vi "Synthetic_Jet_LDA.vi"() -> (5 "Plug in titles":string[](array[string]), 7 "Plug in values":string[](array[string]))   [LabVIEW 2011]
uses:
  Controls/SJ_Data_Cluster.ctl
  Controls/SJ_Results_Cluster.ctl
  Controls/SJ_Channels.ctl
  Globals/Meas_global.vi
  <vilib>/Analysis/1siggen.llb/Ramp Pattern by Delta.vi
  <vilib>/Analysis/NI_AALBase.lvlib
  <vilib>/gmath/NI_Gmath.lvlib
  <vilib>/Analysis/NI_AALPro.lvlib
panel:
  out "Data Array":dbl[][](array[numeric])
  out "ALL filepath":path
  out "File Paths":path[][](array[path])
  out "Channel Varaibles":string[](array[string])
  out "Variable Names":string[](array[string])
  out "Target Frequency":dbl
  out "Results Folder Exists?":bool
  out "SJ Results Array":T1[](array[typedef])
  out "Dwell Time":u32=200
  out "No of Analogue Samples":i32=40000
  out "Analogue Aquisition Time":dbl=999.975
  out "Analogue Samples":i32=39999
  out "dt":dbl=inf
  out "No of bins":i32
  out "Analogue Fs":dbl=40000.0
  out "Next Frequency":dbl=1060.0
  out "Zero Values":dbl[](array[numeric])=[0.0030001498508715582, 0.0061511235517187676, 2.208881239967972, 0.0008108304920773175, 1.5203627177178738]
  out "SJ Data":T2={"Do"=0.005, "Dc"=0.038, "Ho"=0.01, "Hc"=0.008, "K"=1.14, "beta"=0.424, "Vc"=2.0, "Vo"=2.375}
  out "Current Frequency":dbl=1039.7638647645044 format="%0.4f"
  out "Frequency Array":dbl[](array[numeric])=[600.0, 620.0, 640.0, 660.0, 680.0, 700.0, 720.0, 740.0, 760.0, 780.0, 800.0, 820.0, 840.0, 860.0, 880.0, 900.0, 920.0, 940.0, 960.0, 980.0, 1000.0, 1020.0, 1040.0, 1060.0, 1080.0, 1100.0, 1120.0, 1140.0, 1160.0, 1180.0, 1200.0]
  # "You Must have selected the \"Save Data\" option on the \nMeasurement Program for this vi to work correctly"
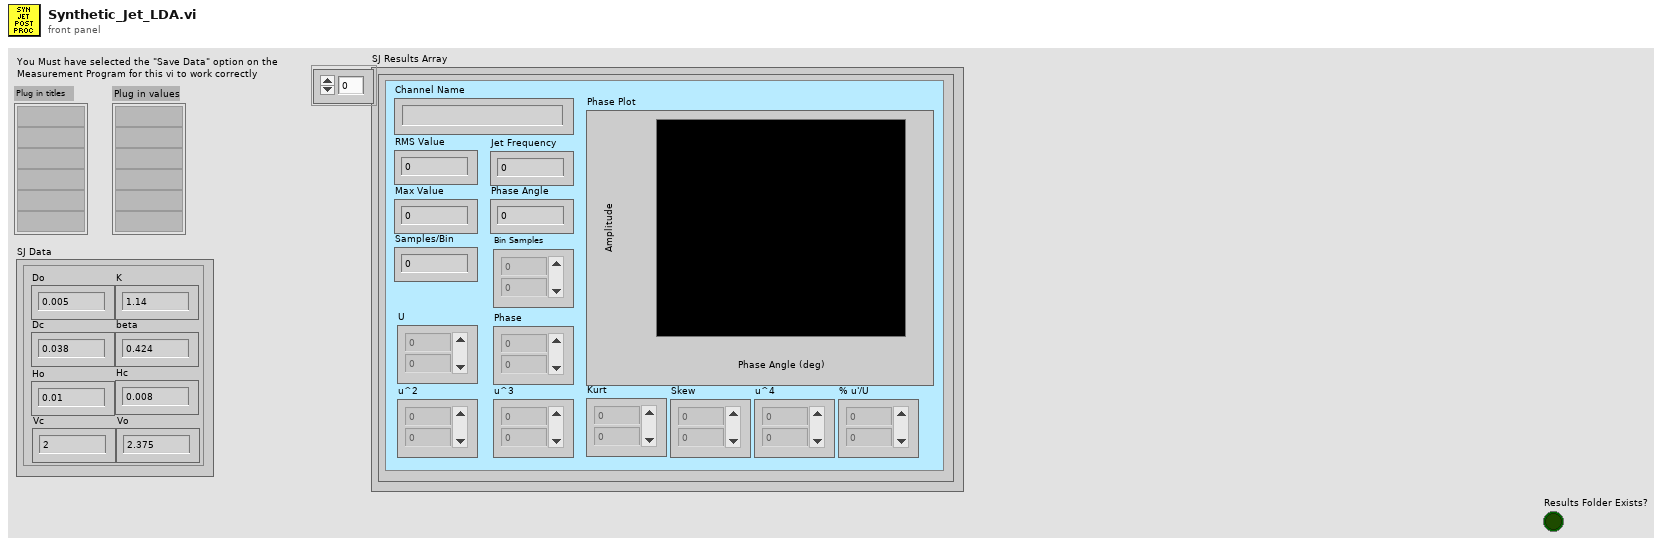
[diagram p1: front panel]
types:
  T1 = typedef "SJ_Results_Cluster.ctl" = cluster{"U":dbl[], "u^2":dbl[], "u^3":dbl[], "u^4":dbl[], "Skew":dbl[], "Kurt":dbl[], "% u'/U":dbl[], "Phase":dbl[], "Bin Samples":dbl[], "Phase Plot":cluster{"Phase Angle":dbl[], dbl[]}, "Channel Name":string, "Max Value":dbl, "RMS Value":dbl, "Phase Angle":dbl, "Jet Frequency":dbl, "Samples/Bin":i32}
  T2 = typedef "SJ_Data_Cluster.ctl" = cluster{"Do":dbl, "Dc":dbl, "Ho":dbl, "Hc":dbl, "K":dbl, "beta":dbl, "Vc":dbl, "Vo":dbl}
  T3 = typedef "SJ_Channels.ctl" = string[]
  T4 = typedef "Analysis_info_cluster.ctl" = cluster{"Colour":u32, "Inst type":T5, "Inst name":string, "Symbol":string, "Code name":string, "Extra Info":string, "Inst Array":T6, "Index":i32, "Voltage Index":i32, "Extra Titles":string[], "Extra Values":string[], "Eng Values":dbl[], "Time (ms)":dbl[], "TT / Voltage":dbl[], "U":dbl, "u^2":dbl, "u^3":dbl, "u^4":dbl, "Skew_u":dbl, "Kurt_u":dbl, "Mean % Err":dbl, "% u'/U":dbl}
  T5 = typedef "Inst_type.ctl" = enum16{"Propeller anemometer", "Raw voltage", "Pressure Transducer", "Pitot-static tube", "Preston tube", "Hot wire", "Cross wire 1", "Cross wire 2", "Generic Linear", "Generic Polynomial", "Generic BackPoly", "Fast FID", "Thermocouple", "Cold wire", "Pulsed Wire", "LDA Vel", "LDA Tran time", "LDA Arr time"}
  T6 = typedef "Instrument_Array.ctl" = enum16{"PWA", "LDA", "Analogue"}
  T7 = typedef "Post_Process.ctl" = enum16{"Take New Data", "Post Process Raw Data File"}
  T8 = cluster{"Name":string, "X":dbl, "Y":dbl, "Z":dbl}[]
  T9 = cluster{"Name":string, "X":dbl, "Y":dbl, "Z":dbl}
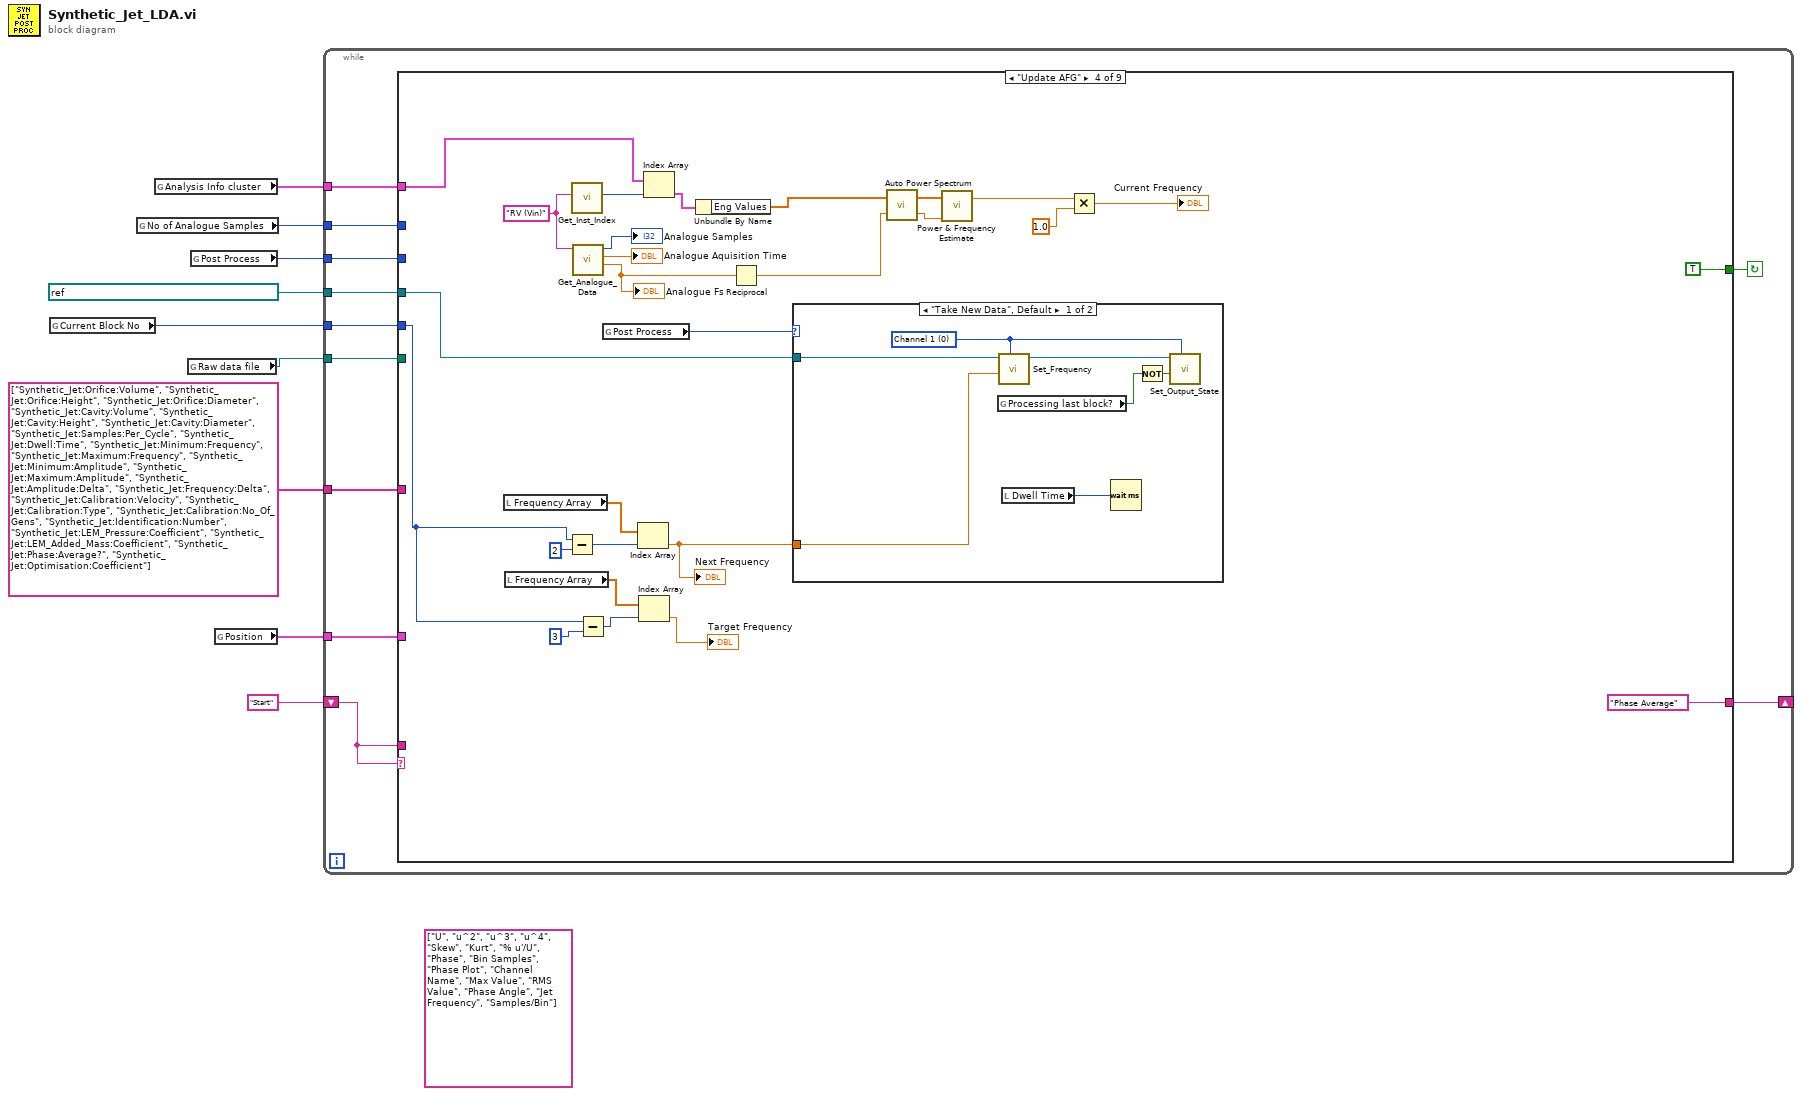
[diagram p0: block diagram]
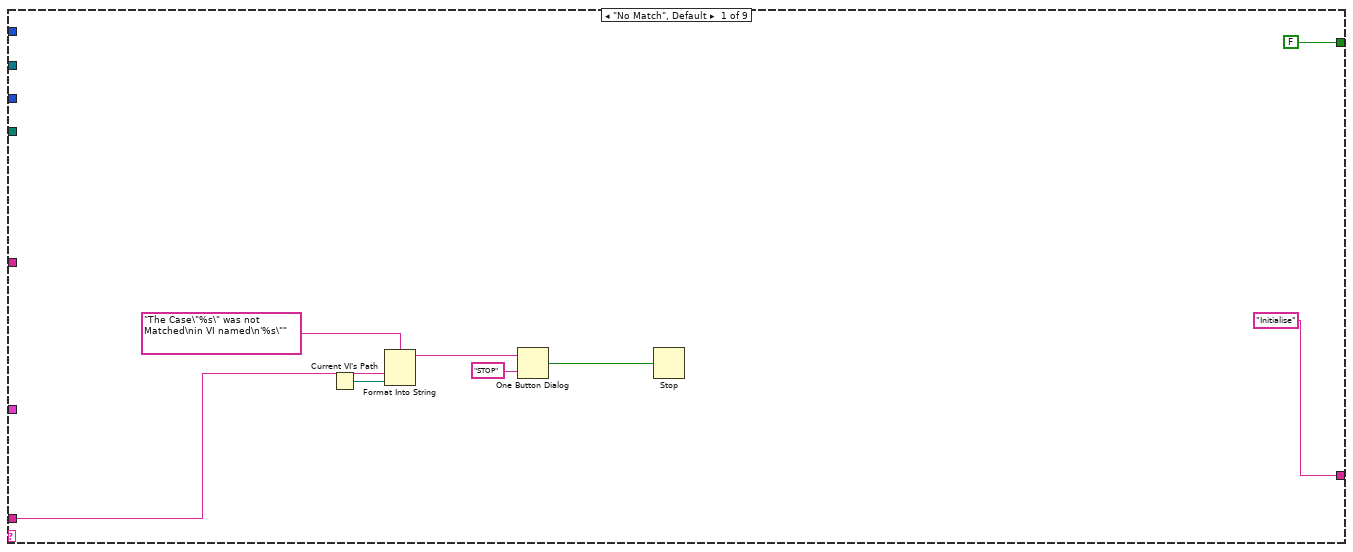
[diagram p2: hidden frame]
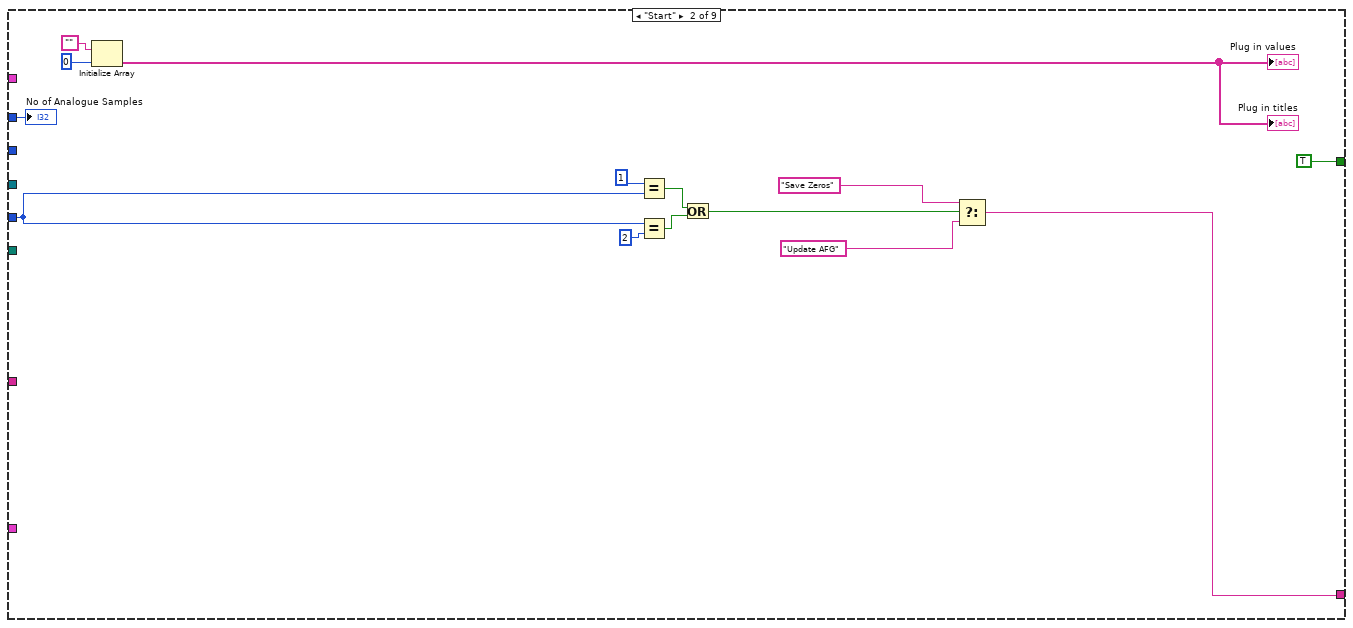
[diagram p3: hidden frame]
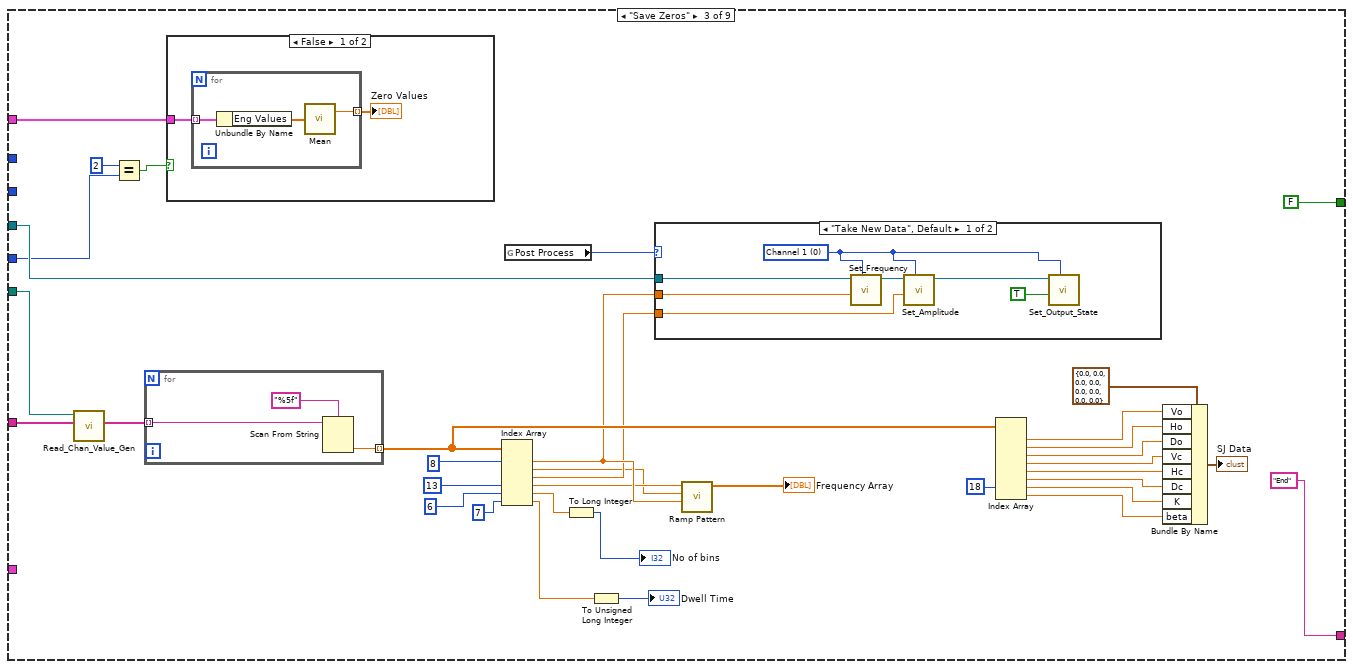
[diagram p4: hidden frame]
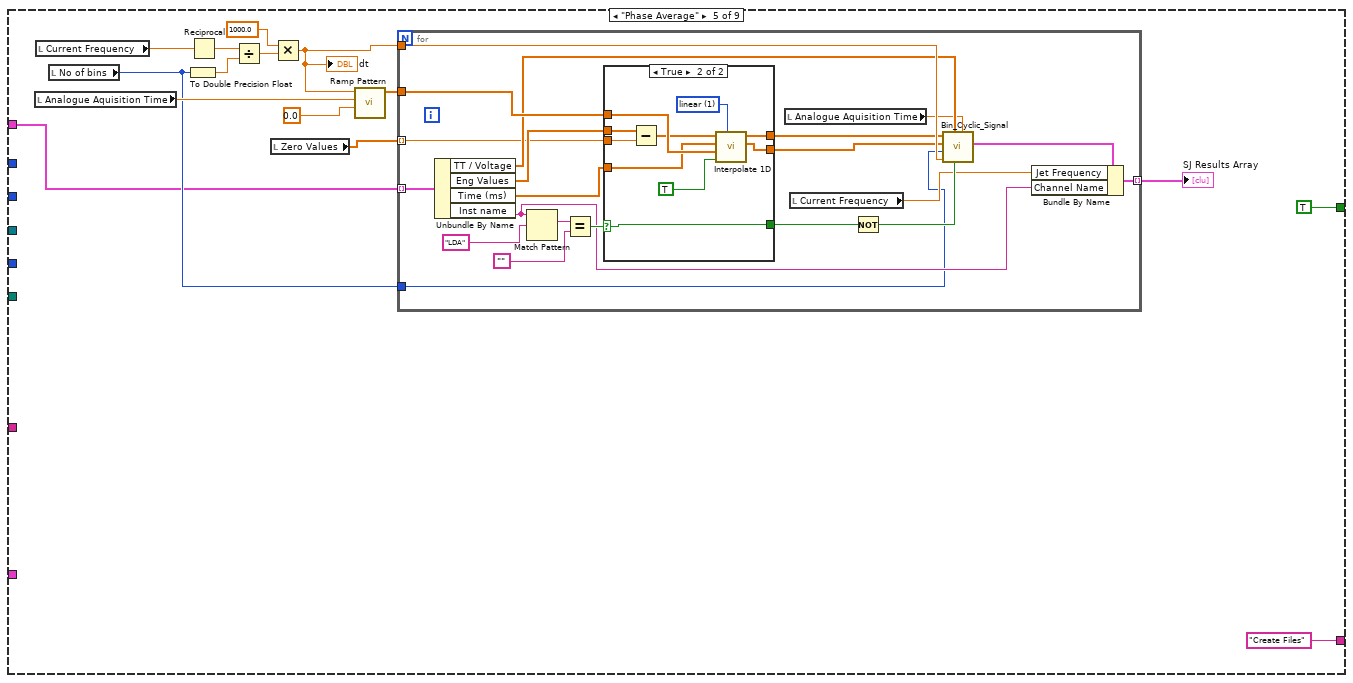
[diagram p8: hidden frame]
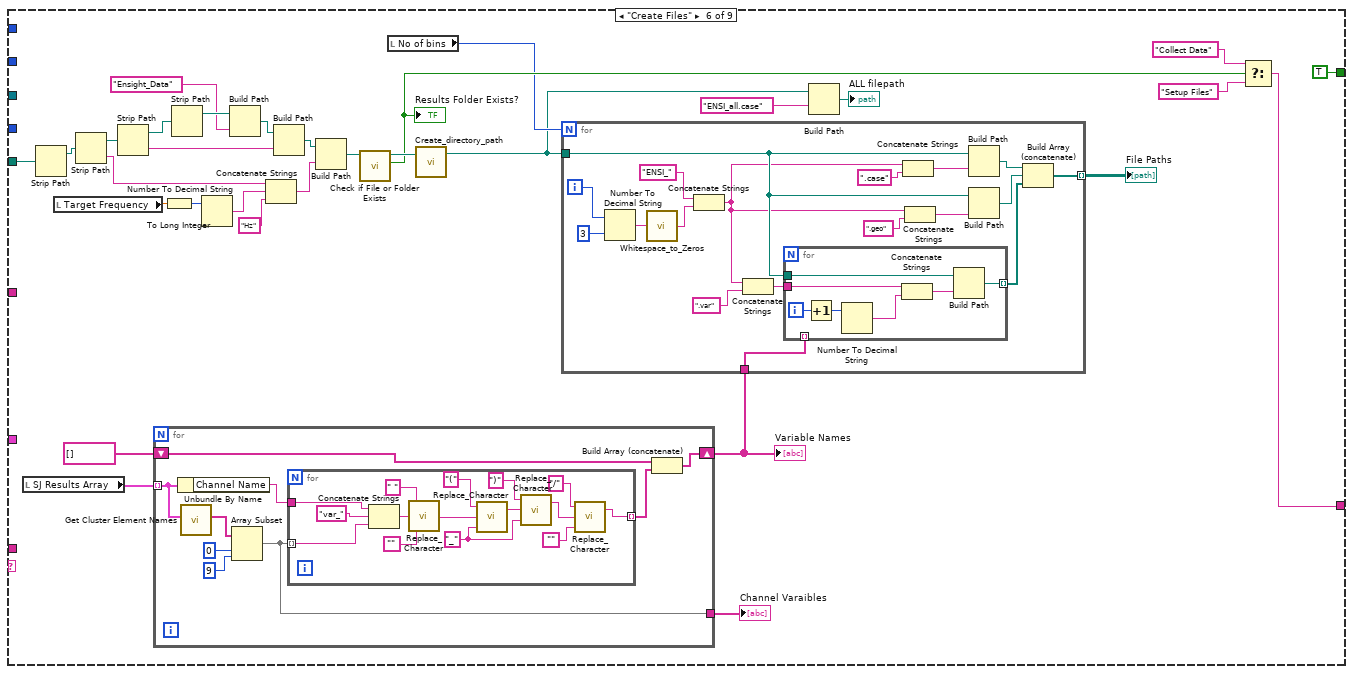
[diagram p10: hidden frame]
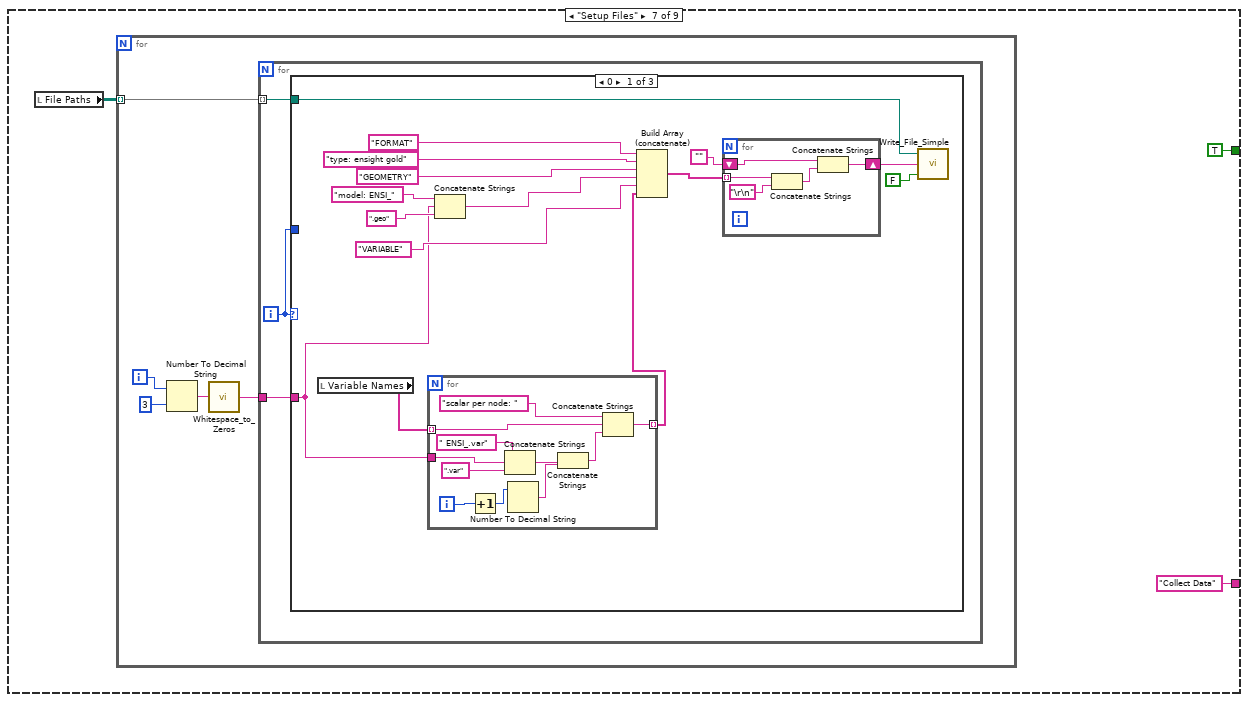
[diagram p11: hidden frame]
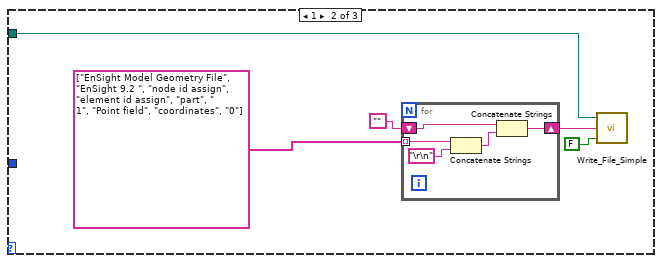
[diagram p12: hidden frame]
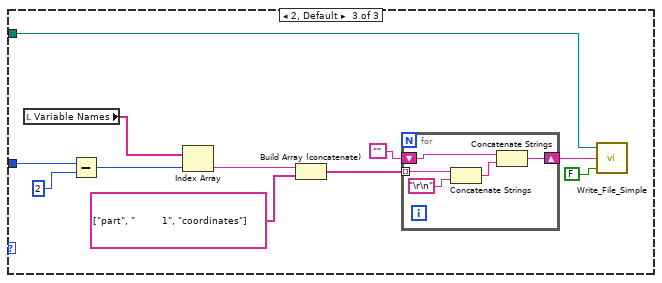
[diagram p13: hidden frame]
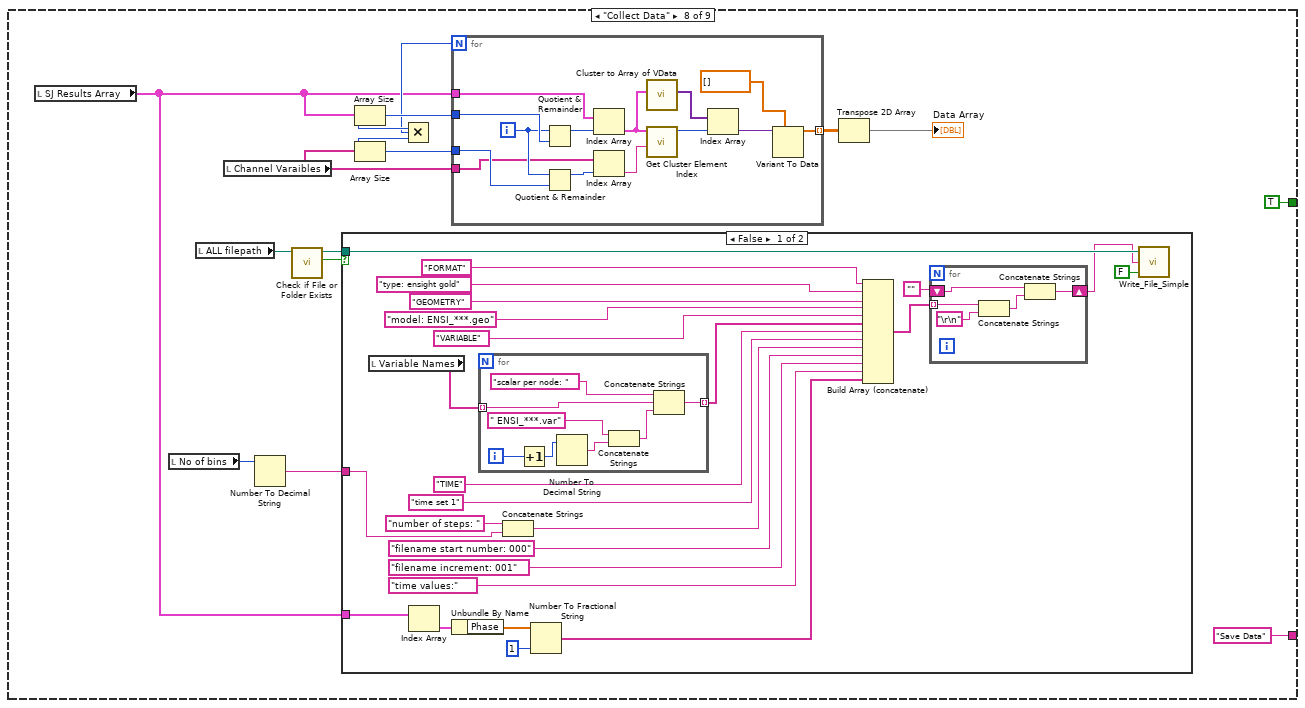
[diagram p14: hidden frame]
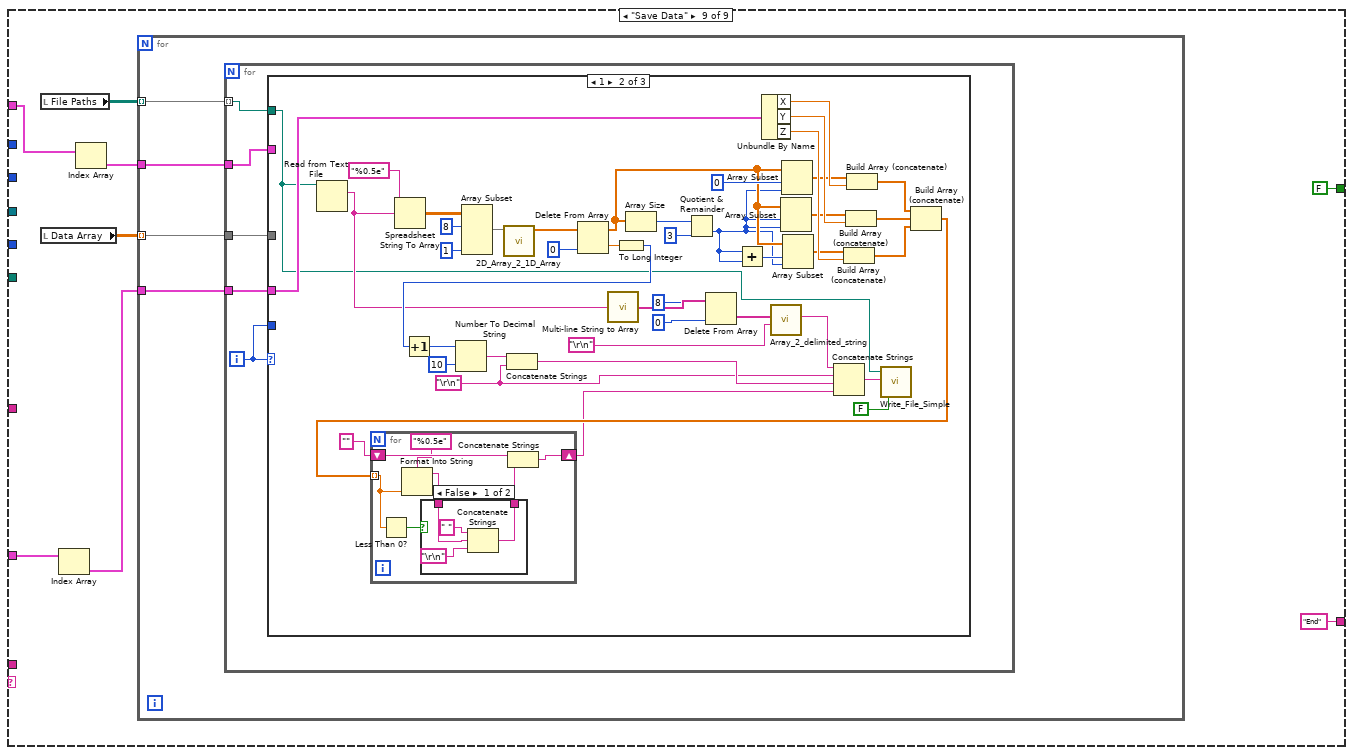
[diagram p16: hidden frame]
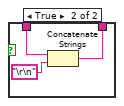
[diagram p18: hidden frame]
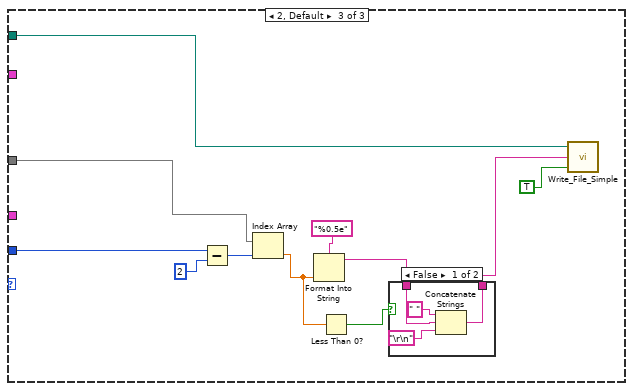
[diagram p19: hidden frame]
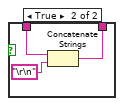
[diagram p20: hidden frame]
diagram:
  (unwired) string[] ["U", "u^2", "u^3", "u^4", "Skew", "Kurt", "% u'/U", "Phase", "Bin Samples", "Phase Plot", "Channel Name", "Max Value", "RMS Value", "Phase Angle", "Jet Frequency", "Samples/Bin"] ("Element Names")
  n1 = global read "Meas_global.vi" "Current Block No"() -> (w7:i32)
  n2 = global read "Meas_global.vi" "No of Analogue Samples"() -> (w5:i32)
  n3 = global read "Meas_global.vi" "Analysis Info cluster"() -> (w6:T4[])
  n4 = global read "Meas_global.vi" "Raw data file"() -> (w8:path)
  n5 = global read "Meas_global.vi" "Post Process"() -> (w3:T7)
  n6 = global read "Meas_global.vi" "Position"() -> (w4:T8)
  n7 = while {
    shift-left: "Start" -> [w20]
    shift-right: [w14] -> _
    tunnel: w8 -> [w19]
    tunnel: w7 -> [w15]
    tunnel: w6 -> [w18]
    tunnel: w5 -> [w17]
    tunnel: w4 -> [w16]
    tunnel: w3 -> [w12]
    tunnel: T3 ["Synthetic_Jet:Orifice:Volume", "Synthetic_Jet:Orifice:Height", "Synthetic_Jet:Orifice:Diameter", "Synthetic_Jet:Cavity:Volume", "Synthetic_Jet:Cavity:Height", "Synthetic_Jet:Cavity:Diameter", "Synthetic_Jet:Samples:Per_Cycle", "Synthetic_Jet:Dwell:Time", "Synthetic_Jet:Minimum:Frequency", "Synthetic_Jet:Maximum:Frequency", "Synthetic_Jet:Minimum:Amplitude", "Synthetic_Jet:Maximum:Amplitude", "Synthetic_Jet:Amplitude:Delta", "Synthetic_Jet:Frequency:Delta", "Synthetic_Jet:Calibration:Velocity", "Synthetic_Jet:Calibration:Type", "Synthetic_Jet:Calibration:No_Of_Gens", "Synthetic_Jet:Identification:Number", "Synthetic_Jet:LEM_Pressure:Coefficient", "Synthetic_Jet:LEM_Added_Mass:Coefficient", "Synthetic_Jet:Phase:Average?", "Synthetic_Jet:Optimisation:Coefficient"] ("Synthetic Jet Specific Channels") -> [w11]
    tunnel: refnum<visa-resource-name> "USB0::0x0699::0x0347::C036837::INSTR" ("VISA resource name") -> [w10]
    stop <- w13 continue-if-true
    n8 = case shown="\"Update AFG\"" w20 {
      tunnel: w20 -> [w24 _ _ _ _ _ _ _ _]
      tunnel: w19 -> [_ _ w75 _ _ w196 _ _ _]
      tunnel: w15 -> [_ w34 w52 w103 _ _ _ _ _]
      tunnel: w18 -> [_ _ w54 w111 w130 _ _ _ w392]
      tunnel: w17 -> [_ w29 _ _ _ _ _ _ _]
      tunnel: w16 -> [_ _ _ _ _ _ _ _ w395]
      tunnel: ["Initialise" w39 "End" ("t") "Phase Average" ("t") "Create Files" ("t") w183 "Collect Data" ("t") "Save Data" ("t") "End" ("t")] -> w14
      tunnel: [FALSE TRUE FALSE TRUE TRUE TRUE TRUE TRUE FALSE] -> w13
      tunnel: w12 -> [_ _ _ _ _ _ _ _ _]
      tunnel: w11 -> [_ _ w74 _ _ _ _ _ _]
      tunnel: w10 -> [_ _ w60 w114 _ _ _ _ _]
      frame "No Match", Default {
        n9 = Current VI's Path() -> (path=w23:path)
        n10 = Format Into String(format string="The Case\"%s\" was not Matched\nin VI named\n'%s\"" ("Format String"), w24, w23) -> (resulting string=w27:string)  [unwired: 2 in, 1 out]
        n11 = One Button Dialog(message=w27, button name ("OK")="STOP") -> (true=w25:bool)
        n12 = Stop(stop? (T)=w25) -> ()
      }
      frame "Start" {
        n13 = Initialize Array("", 0) -> (→"Plug in values" →"Plug in titles":string[])
        n14 = Equal?(x=1, y=w34) -> (x = y?=w32:bool)
        n15 = Equal?(x=w34, y=2 ("x")) -> (x = y?=w33:bool)
        n16 = Or(x=w32, y=w33) -> (x .or. y?=w31:bool)
        n17 = Select(t="Save Zeros", s=w31, f="Update AFG") -> (s? t:f=w39:string)
        "No of Analogue Samples" <- w29
      }
      frame "Save Zeros" {
        n18 = call "Read_Chan_Value_Gen.vi"("Desired Ch Names"=w74, "Raw data file"=w75) -> ("Values"=w64:string[])  [unwired: 9 in]
        n19 = Equal?(x=2, y=w52) -> (x = y?=w50:bool)
        n20 = for {
          tunnel: w64 -> [w93] mode=indexing
          tunnel: [w91] -> w59 mode=indexing
          n21 = Scan From String(format string="%5f", input string=w93) -> (output 1=w91:dbl)  [unwired: 3 in, 3 out]
        }
        n22 = case shown="False" w50 {
          tunnel: w54 -> [w80 _]
          frame False {
            n23 = for {
              tunnel: w80 -> [w83] mode=indexing
              tunnel: [w81] -> w79 mode=indexing
              n24 = Unbundle By Name(w83) -> ("Eng Values"=w82:dbl[])
              n25 = call <vilib>:"Mean.vi"("X"=w82) -> ("mean"=w81:dbl)  [unwired: 1 out]
            }
            "Zero Values" <- w79
          }
          frame True {
          }
        }
        n26 = Index Array(array=w59, index #1=8 ("index"), index #4=13 ("index"), index #5=6 ("index"), index #6=7 ("index")) -> (element #1=w58:dbl, element #2=w49:dbl, element #3=w57:dbl, element #4=w56:dbl, element #5=w47:dbl, element #6=w45:dbl)  [unwired: 2 in]
        n27 = global read "Meas_global.vi" "Post Process"() -> (w61:T7)
        n28 = To Long Integer(number=w47) -> (32bit integer=→"No of bins":i32)
        n29 = To Unsigned Long Integer(number=w45) -> (unsigned 32bit integer=→"Dwell Time":u32)
        n30 = case shown="\"Take New Data\", Default" w61 {
          tunnel: w57 -> [w90 _]
          tunnel: w58 -> [w85 _]
          tunnel: w60 -> [w84 _]
          frame "Take New Data", Default {
            w87 = u16 0 items=["Channel 1", "Channel 2"] ("Menu Ring")
            n31 = call "Set_Frequency.vi"("Menu Ring"=w87, "Frequency"=w85, "VISA resource name"=w84) -> ("VISA resource name out"=w88:refnum<visa-resource-name>)  [unwired: 8 in]
            n32 = call "Set_Amplitude.vi"("Menu Ring 2"=w87, "Amplitude"=w90, "VISA resource name"=w88) -> ("VISA resource name out"=w89:refnum<visa-resource-name>)  [unwired: 8 in]
            n33 = call "Set_Output_State.vi"("Menu Ring"=w87, "Output State"=TRUE, "VISA resource name"=w89) -> ()  [unwired: 9 in]
          }
          frame "Post Process Raw Data File" {
          }
        }
        n34 = call-poly <vilib>:"Ramp Pattern.vi"("start"=w58, "end"=w49, "delta"=w56) -> ("Ramp Pattern"=→"Frequency Array":dbl[])  [unwired: 6 in, 2 out]
        n35 = Index Array(array=w59, index #7=18 ("index")) -> (element #1=w73:dbl, element #2=w72:dbl, element #3=w71:dbl, element #4=w70:dbl, element #5=w69:dbl, element #6=w68:dbl, element #7=w66:dbl, element #8=w65:dbl)  [unwired: 7 in]
        n36 = Bundle By Name(cluster=T2 {"Do"=0.0, "Dc"=0.0, "Ho"=0.0, "Hc"=0.0, "K"=0.0, "beta"=0.0, "Vc"=0.0, "Vo"=0.0} ("SJ_Data_Cluster"), "Vo"=w73, "Ho"=w72, "Do"=w71, "Vc"=w70, "Hc"=w69, "Dc"=w68, "K"=w66, "beta"=w65) -> (→"SJ Data":T2)
      }
      frame "Update AFG" {
        w112 = "RV (Vin)" ("Inst name search")
        n37 = local read "Frequency Array"() -> (w119:dbl[])
        n38 = local read "Frequency Array"() -> (w104:dbl[])
        n39 = Subtract(x=w103, y=2) -> (x-y=w118:i32)
        n40 = call "Get_Inst_Index.vi"("Inst name search"=w112) -> ("Index of Instance"=w110:i32)  [unwired: 8 in, 2 out]
        n41 = call "Get_Analogue_Data.vi"("Inst (Inst 2 if blank)"=w112) -> ("Analogue Fs"=w96:dbl, "Analogue Aquasition Time"=→"Analogue Aquisition Time":dbl, "Analogue Samples"=→"Analogue Samples":i32)  [unwired: 8 in]
        "Analogue Fs" <- w96
        n42 = Subtract(x=w103, y=3) -> (x-y=w101:i32)
        n43 = global read "Meas_global.vi" "Post Process"() -> (w115:T7)
        n44 = Index Array(array=w119, index=w118) -> (element=w116:dbl)
        "Next Frequency" <- w116
        n45 = Index Array(array=w104, index=w101) -> (element=→"Target Frequency":dbl)
        n46 = Index Array(array=w111, index=w110) -> (element=w109:T4)
        n47 = Unbundle By Name(w109) -> ("Eng Values"=w94:dbl[])
        n48 = Reciprocal(x=w96) -> (1/x=w95:dbl)
        n49 = case shown="\"Take New Data\", Default" w115 {
          tunnel: w116 -> [w126 _]
          tunnel: w114 -> [w124 _]
          frame "Take New Data", Default {
            w127 = u16 0 items=["Channel 1", "Channel 2"] ("Menu Ring")
            n50 = global read "Meas_global.vi" "Processing last block?"() -> (w122:bool)
            n51 = call "Set_Frequency.vi"("Menu Ring"=w127, "Frequency"=w126, "VISA resource name"=w124) -> ("VISA resource name out"=w125:refnum<visa-resource-name>)  [unwired: 8 in]
            n52 = local read "Dwell Time"() -> (w121:u32)
            n53 = Wait (ms)(milliseconds to wait=w121) -> ()  [unwired: 1 out]
            n54 = Not(x=w122) -> (.not. x?=w123:bool)
            n55 = call "Set_Output_State.vi"("Menu Ring"=w127, "Output State"=w123, "VISA resource name"=w125) -> ()  [unwired: 9 in]
          }
          frame "Post Process Raw Data File" {
          }
        }
        n56 = call <vilib>:"Auto Power Spectrum.vi"("dt"=w95, "Signal (V)"=w94) -> ("df"=w98:dbl, "Power Spectrum (V^2 rms)"=w97:dbl[])
        n57 = call <vilib>:"Power & Frequency Estimate.vi"("df"=w98, "Power Spectrum (V^2 rms)"=w97) -> ("est frequency peak"=w99:dbl)  [unwired: 4 in, 1 out]
        n58 = Multiply(x=w99, y=1.0) -> (x*y=→"Current Frequency":dbl)
      }
      frame "Phase Average" {
        n59 = local read "Analogue Aquisition Time"() -> (w137:dbl)
        n60 = local read "Current Frequency"() -> (w134:dbl)
        n61 = local read "No of bins"() -> (w131:i32)
        n62 = To Double Precision Float(number=w131) -> (double precision float=w140:dbl)
        n63 = Reciprocal(x=w134) -> (1/x=w139:dbl)
        n64 = Divide(x=w139, y=w140) -> (x/y=w136:dbl)
        n65 = local read "Zero Values"() -> (w129:dbl[])
        n66 = Multiply(x=1000.0, y=w136) -> (x*y=w132:dbl)
        "dt" <- w132
        n67 = call-poly <vilib>:"Ramp Pattern.vi"("start"=0.0, "end"=w137, "delta"=w132) -> ("Ramp Pattern"=w133:dbl[])  [unwired: 6 in, 2 out]
        n68 = for {
          tunnel: w133 -> [w163]
          tunnel: w132 -> [w162]
          tunnel: w131 -> [w147]
          tunnel: w130 -> [w145] mode=indexing
          tunnel: w129 -> [w144] mode=indexing
          tunnel: [w143] -> w128 mode=indexing
          n69 = Unbundle By Name(w145) -> ("TT / Voltage"=w152:dbl[], "Eng Values"=w156:dbl[], "Time (ms)"=w157:dbl[], "Inst name"=w149:string)
          n70 = Match Pattern(string=w149, regular expression="LDA") -> (match substring=w160:string)  [unwired: 1 in, 3 out]
          n71 = Equal?(x=w160, y="") -> (x = y?=w158:bool)
          n72 = case shown="True" w158 {
            selector: w158 -> [w164 w170]
            tunnel: w163 -> [_ w175]
            tunnel: w157 -> [w165 w174]
            tunnel: w156 -> [w166 w169]
            tunnel: [w166 w172] -> w146
            tunnel: [w165 w171] -> w155
            tunnel: [w164 w170] -> w154
            tunnel: w144 -> [_ w167]
            frame False {
            }
            frame True {
              w176 = 1 items=["nearest", "linear", "spline", "cubic Hermite", "Lagrange"] ("method")
              n73 = Subtract(x=w169, y=w167) -> (x-y=w168:dbl[])
              n74 = call <vilib>:"Interpolate 1D.vi"("method"=w176, "X is monotonic"=TRUE, "xi"=w175, "X"=w174, "Y"=w168) -> ("xi used"=w171:dbl[], "yi"=w172:dbl[])  [unwired: 4 in, 1 out]
            }
          }
          n75 = local read "Analogue Aquisition Time"() -> (w151:dbl)
          n76 = local read "Current Frequency"() -> (w148:dbl)
          n77 = Not(x=w154) -> (.not. x?=w153:bool)
          n78 = call "Bin_Cyclic_Signal.vi"("Max Time"=w151, "LDA Data? (False)"=w153, "Transit Time"=w152, "dt"=w162, "No of bins"=w147, "Time"=w155, "Eng Values"=w146) -> ("SJ Results"=w150:T1)  [unwired: 4 in]
          n79 = Bundle By Name(cluster=w150, "Jet Frequency"=w148, "Channel Name"=w149) -> (w143:T1)
        }
        "SJ Results Array" <- w128
      }
      frame "Create Files" {
        n80 = local read "SJ Results Array"() -> (w179:T1[])
        n81 = Strip Path(path=w196) -> (stripped path=w206:path)  [unwired: 1 out]
        n82 = local read "Target Frequency"() -> (w195:dbl)
        n83 = Strip Path(path=w206) -> (stripped path=w205:path, name=w193:string)
        n84 = Strip Path(path=w205) -> (stripped path=w204:path, name=w200:string)
        n85 = for {
          tunnel: w179 -> [w233] mode=indexing
          shift-right: [w237] -> w188
          shift-left: string[] [] -> [w235]
          tunnel: [w234] -> w187
          n86 = Unbundle By Name(w233) -> ("Channel Name"=w238:string)
          n87 = call "Get Cluster Element Names.vi"("Cluster"=w233) -> ("Element Names"=w241:string[])  [unwired: 9 in, 1 out]
          n88 = Array Subset(array=w241, index=0, length=9) -> (w234:string[])
          n89 = for {
            tunnel: w234 -> [w256] mode=indexing
            tunnel: w238 -> [w255]
            tunnel: [w243] -> w236 mode=indexing
            w247 = "_" ("Replace with")
            n90 = Concatenate Strings(w255, "var_" ("string"), w256) -> (w253:string)
            n91 = call "Replace_Character.vi"("Replace with"="", "Input String"=w253, "Search For"=" ") -> ("Output string"=w242:string)  [unwired: 1 out]
            n92 = call "Replace_Character.vi"("Replace with"=w247, "Input String"=w242, "Search For"="(") -> ("Output string"=w249:string)  [unwired: 1 out]
            n93 = call "Replace_Character.vi"("Replace with"=w247, "Input String"=w249, "Search For"=")") -> ("Output string"=w246:string)  [unwired: 1 out]
            n94 = call "Replace_Character.vi"("Replace with"="", "Input String"=w246, "Search For"="/") -> ("Output string"=w243:string)  [unwired: 1 out]
          }
          n95 = Build Array (concatenate)(w235, w236) -> (w237:string[])
        }
        "Variable Names" <- w188
        "Channel Varaibles" <- w187
        n96 = To Long Integer(number=w195) -> (32bit integer=w194:i32)
        n97 = Strip Path(path=w204) -> (stripped path=w203:path)  [unwired: 1 out]
        n98 = Number To Decimal String(number=w194) -> (decimal integer string=w192:string)  [unwired: 1 in]
        n99 = Build Path(base path=w203, name or relative path="Ensight_Data") -> (appended path=w201:path)
        n100 = Concatenate Strings(w193, w192, "Hz" ("string")) -> (w190:string)
        n101 = Build Path(base path=w201, name or relative path=w200) -> (appended path=w197:path)
        n102 = Build Path(base path=w197, name or relative path=w190) -> (appended path=w198:path)
        n103 = call <vilib>:"Check if File or Folder Exists.vi"("path"=w198) -> ("file or folder exists?"=w184:bool, "dup path"=w199:path)  [unwired: 8 in, 1 out]
        "Results Folder Exists?" <- w184
        n104 = local read "No of bins"() -> (w182:i32)
        n105 = call "Create_directory_path.vi"("Path name"=w199) -> ("Path name Out"=w177:path)  [unwired: 1 in, 1 out]
        n106 = for {
          N: w182 -> [_]
          tunnel: w177 -> [w225]
          tunnel: w188 -> [w224]
          tunnel: [w223] -> w178 mode=indexing
          i -> [w219]
          n107 = Number To Decimal String(number=w219, width (-)=i16 3) -> (decimal integer string=w217:string)
          n108 = call "Whitespace_to_Zeros.vi"("Input String"=w217) -> ("Output String"=w213:string)  [unwired: 6 in]
          n109 = Concatenate Strings("ENSI_" ("name or relative path"), w213) -> (w209:string)
          n110 = Concatenate Strings(w209, ".var" ("name or relative path")) -> (w208:string)
          n111 = for {
            tunnel: w225 -> [w232]
            tunnel: [w227] -> w220 mode=indexing
            tunnel: w224 -> [_] mode=indexing
            tunnel: w208 -> [w226]
            i -> [w231]
            n112 = Increment(x=w231) -> (x+1=w230:i32)
            n113 = Number To Decimal String(number=w230) -> (decimal integer string=w229:string)  [unwired: 1 in]
            n114 = Concatenate Strings(w226, w229) -> (w228:string)
            n115 = Build Path(base path=w232, name or relative path=w228) -> (appended path=w227:path)
          }
          n116 = Concatenate Strings(w209, ".case" ("name or relative path")) -> (w216:string)
          n117 = Concatenate Strings(w209, ".geo" ("name or relative path")) -> (w212:string)
          n118 = Build Path(base path=w225, name or relative path=w216) -> (appended path=w221:path)
          n119 = Build Path(base path=w225, name or relative path=w212) -> (appended path=w222:path)
          n120 = Build Array (concatenate)(w221, w222, w220) -> (w223:path[])
        }
        "File Paths" <- w178
        n121 = Build Path(base path=w177, name or relative path="ENSI_all.case") -> (appended path=→"ALL filepath":path)
        n122 = Select(t="Collect Data", s=w184, f="Setup Files" ("t")) -> (s? t:f=w183:string)
      }
      frame "Setup Files" {
        n123 = local read "File Paths"() -> (w258:path[][])
        n124 = for {
          tunnel: w258 -> [w264] mode=indexing
          i -> [w261]
          n125 = Number To Decimal String(number=w261, width (-)=i16 3) -> (decimal integer string=w262:string)
          n126 = call "Whitespace_to_Zeros.vi"("Input String"=w262) -> ("Output String"=w260:string)  [unwired: 6 in]
          n127 = for {
            tunnel: w264 -> [w267] mode=indexing
            tunnel: w260 -> [w265]
            i -> [w266]
            n128 = case shown="0" w266 {
              tunnel: w267 -> [w278 w300 w319]
              tunnel: w266 -> [_ _ w314]
              tunnel: w265 -> [w268 _ _]
              frame 0 {
                n129 = local read "Variable Names"() -> (w282:string[])
                n130 = for {
                  tunnel: w282 -> [w294] mode=indexing
                  tunnel: [w292] -> w277 mode=indexing
                  tunnel: w268 -> [w289]
                  i -> [w296]
                  n131 = Increment(x=w296) -> (x+1=w297:i32)
                  n132 = Concatenate Strings(" ENSI_.var", w289, ".var") -> (w291:string)
                  n133 = Number To Decimal String(number=w297) -> (decimal integer string=w295:string)  [unwired: 1 in]
                  n134 = Concatenate Strings(w291, w295) -> (w293:string)
                  n135 = Concatenate Strings("scalar per node: ", w294, w293) -> (w292:string)
                }
                n136 = Concatenate Strings("model: ENSI_", w268, ".geo") -> (w270:string)
                n137 = Build Array (concatenate)("FORMAT", "type: ensight gold", "GEOMETRY", w270, "VARIABLE", w277) -> (w276:string[])
                n138 = for {
                  tunnel: w276 -> [w287] mode=indexing
                  shift-right: [w285] -> w280
                  shift-left: "" -> [w283]
                  n139 = Concatenate Strings(w287, "\r\n") -> (w284:string)
                  n140 = Concatenate Strings(w283, w284) -> (w285:string)
                }
                n141 = call "Write_File_Simple.vi"("append to file? (new file:F)"=FALSE, "character string"=w280, "file path"=w278) -> ()  [unwired: 2 out]
              }
              frame 1 {
                n142 = for {
                  tunnel: string[] ["EnSight Model Geometry File", "EnSight 9.2 ", "node id assign", "element id assign", "part", "         1", "Point field", "coordinates", "0"] -> [w308] mode=indexing
                  shift-right: [w306] -> w302
                  shift-left: "" -> [w304]
                  n143 = Concatenate Strings(w308, "\r\n") -> (w305:string)
                  n144 = Concatenate Strings(w304, w305) -> (w306:string)
                }
                n145 = call "Write_File_Simple.vi"("append to file? (new file:F)"=FALSE, "character string"=w302, "file path"=w300) -> ()  [unwired: 2 out]
              }
              frame 2, Default {
                n146 = local read "Variable Names"() -> (w315:string[])
                n147 = Subtract(x=w314, y=2) -> (x-y=w312:i32)
                n148 = Index Array(array=w315, index=w312) -> (element=w311:string)
                n149 = Build Array (concatenate)(w311, string[] ["part", "         1", "coordinates"]) -> (w309:string[])
                n150 = for {
                  tunnel: w309 -> [w324] mode=indexing
                  shift-right: [w322] -> w317
                  shift-left: "" -> [w320]
                  n151 = Concatenate Strings(w324, "\r\n") -> (w321:string)
                  n152 = Concatenate Strings(w320, w321) -> (w322:string)
                }
                n153 = call "Write_File_Simple.vi"("append to file? (new file:F)"=FALSE, "character string"=w317, "file path"=w319) -> ()  [unwired: 2 out]
              }
            }
          }
        }
      }
      frame "Collect Data" {
        n154 = local read "SJ Results Array"() -> (w327:T1[])
        n155 = local read "No of bins"() -> (w326:i32)
        n156 = local read "ALL filepath"() -> (w330:path)
        n157 = local read "Channel Varaibles"() -> (w335:string[])
        n158 = Number To Decimal String(number=w326) -> (decimal integer string=w325:string)  [unwired: 1 in]
        n159 = call <vilib>:"Check if File or Folder Exists.vi"("path"=w330) -> ("file or folder exists?"=w329:bool, "dup path"=w328:path)  [unwired: 8 in, 1 out]
        n160 = case shown="False" w329 {
          tunnel: w328 -> [w363 _]
          tunnel: w327 -> [w361 _]
          tunnel: w325 -> [w345 _]
          frame False {
            n161 = local read "Variable Names"() -> (w352:string[])
            n162 = Index Array(array=w361) -> (element=w360:T1)  [unwired: 1 in]
            n163 = Unbundle By Name(w360) -> ("Phase"=w359:dbl[])
            n164 = for {
              tunnel: w352 -> [w372] mode=indexing
              tunnel: [w370] -> w351 mode=indexing
              i -> [w374]
              n165 = Increment(x=w374) -> (x+1=w375:i32)
              n166 = Number To Decimal String(number=w375) -> (decimal integer string=w373:string)  [unwired: 1 in]
              n167 = Concatenate Strings(" ENSI_***.var", w373) -> (w371:string)
              n168 = Concatenate Strings("scalar per node: ", w372, w371) -> (w370:string)
            }
            n169 = Concatenate Strings("number of steps: ", w345) -> (w343:string)
            n170 = Number To Fractional String(number=w359, precision (6)=i16 1) -> (F-format string=w339:string[])  [unwired: 2 in]
            n171 = Build Array (concatenate)("FORMAT", "type: ensight gold", "GEOMETRY", "model: ENSI_***.geo", "VARIABLE", w351, "TIME", "time set 1", w343, "filename start number: 000", "filename increment: 001", "time values:", w339) -> (w348:string[])
            n172 = for {
              tunnel: w348 -> [w368] mode=indexing
              shift-right: [w366] -> w349
              shift-left: "" -> [w364]
              n173 = Concatenate Strings(w368, "\r\n") -> (w365:string)
              n174 = Concatenate Strings(w364, w365) -> (w366:string)
            }
            n175 = call "Write_File_Simple.vi"("append to file? (new file:F)"=FALSE, "character string"=w349, "file path"=w363) -> ()  [unwired: 2 out]
          }
          frame True {
          }
        }
        n176 = Array Size(array=w327) -> (size(s)=w337:i32)
        n177 = Array Size(array=w335) -> (size(s)=w336:i32)
        n178 = Multiply(x=w337, y=w336) -> (x*y=w334:i32)
        n179 = for {
          N: w334 -> [_]
          tunnel: w327 -> [w386]
          tunnel: w337 -> [w385]
          tunnel: w336 -> [w382]
          tunnel: w335 -> [w379]
          tunnel: [w377] -> w333 mode=indexing
          i -> [w381]
          n180 = Quotient & Remainder(x=w381, y=w385) -> (x-y*floor(x/y)=w384:i32)  [unwired: 1 out]
          n181 = Quotient & Remainder(x=w381, y=w382) -> (x-y*floor(x/y)=w380:i32)  [unwired: 1 out]
          n182 = Index Array(array=w386, index=w384) -> (element=w383:T1)
          n183 = Index Array(array=w379, index=w380) -> (element=w378:string)
          n184 = call "Cluster to Array of VData.vi"("Cluster"=w383) -> ("Array of VData"=w388:variant[])  [unwired: 9 in, 1 out]
          n185 = call "Get Cluster Element Index.vi"("Element Name"=w378, "Cluster"=w383) -> ("Element Index"=w387:i32)  [unwired: 9 in]
          n186 = Index Array(array=w388, index=w387) -> (element=w389:variant)
          n187 = Variant To Data(type=dbl[] [], Variant=w389) -> (data=w377:dbl[])  [unwired: 1 in, 1 out]
        }
        n188 = Transpose 2D Array(2D array=w333) -> (transposed array=→"Data Array":dbl[][])
      }
      frame "Save Data" {
        n189 = local read "File Paths"() -> (w396:path[][])
        n190 = local read "Data Array"() -> (w393:dbl[][])
        n191 = Index Array(array=w395) -> (element=w394:T9)  [unwired: 1 in]
        n192 = Index Array(array=w392) -> (element=w391:T4)  [unwired: 1 in]
        n193 = for {
          tunnel: w396 -> [w402] mode=indexing
          tunnel: w394 -> [w401]
          tunnel: w393 -> [w400] mode=indexing
          tunnel: w391 -> [w399]
          n194 = for {
            tunnel: w402 -> [w407] mode=indexing
            tunnel: w401 -> [w406]
            tunnel: w400 -> [w404]
            tunnel: w399 -> [w403]
            i -> [w405]
            n195 = case shown="1" w405 {
              tunnel: w407 -> [_ w408 w475]
              tunnel: w406 -> [_ w444 _]
              tunnel: w405 -> [_ _ w474]
              tunnel: w404 -> [_ _ w465]
              tunnel: w403 -> [_ _ _]
              frame 0 {
              }
              frame 1 {
                w426 = "\r\n"
                n196 = Read from Text File(file (use dialog)=w408) -> (text=w441:string)  [unwired: 3 in, 3 out]
                n197 = Spreadsheet String To Array(format string="%0.5e", spreadsheet string=w441) -> (array=w445:dbl[][])  [unwired: 2 in]
                n198 = Array Subset(array=w445, index (row)=8 ("index"), length (col)=1 ("length")) -> (w448:dbl[][])  [unwired: 2 in]
                n199 = call "2D_Array_2_1D_Array.vi"("Array in"=w448) -> ("Array out"=w449:dbl[])  [unwired: 10 in]
                n200 = Delete From Array(array=w449, index=0) -> (deleted portion=w422:dbl, array with subset deleted=w414:dbl[])  [unwired: 1 in]
                n201 = call "Multi-line String to Array.vi"("Multi lined string"=w441) -> ("Array of string lines"=w440:string[])
                n202 = To Long Integer(number=w422) -> (32bit integer=w443:i32)
                n203 = Increment(x=w443) -> (x+1=w437:i32)
                n204 = Number To Decimal String(number=w437, width (-)=i16 10) -> (decimal integer string=w436:string)
                n205 = Concatenate Strings(w436, w426) -> (w427:string)
                n206 = Array Size(array=w414) -> (size(s)=w417:i32)
                n207 = Quotient & Remainder(x=w417, y=3) -> (floor(x/y)=w412:i32)  [unwired: 1 out]
                n208 = Delete From Array(array=w440, length=8 ("index"), index=0) -> (deleted portion=w424:string[])  [unwired: 1 out]
                n209 = Add(x=w412, y=w412) -> (x+y=w413:i32)
                n210 = Unbundle By Name(w444) -> ("X"=w433:dbl, "Y"=w432:dbl, "Z"=w431:dbl)
                n211 = call "Array_2_delimited_string.vi"("delimiter (Tab)"="\r\n", "Array of Strings"=w424) -> ("delimited string"=w423:string)  [unwired: 9 in]
                n212 = Array Subset(array=w414, index=w412, length=w412) -> (w410:dbl[])
                n213 = Array Subset(array=w414, index=0, length=w412) -> (w411:dbl[])
                n214 = Array Subset(array=w414, index=w413, length=w412) -> (w409:dbl[])
                n215 = Build Array (concatenate)(w409, w431) -> (w428:dbl[])
                n216 = Build Array (concatenate)(w410, w432) -> (w429:dbl[])
                n217 = Build Array (concatenate)(w411, w433) -> (w430:dbl[])
                n218 = Build Array (concatenate)(w430, w429, w428) -> (w421:dbl[])
                n219 = for {
                  tunnel: w421 -> [w452] mode=indexing
                  shift-right: [w457] -> w419
                  shift-left: "" -> [w456]
                  n220 = Less Than 0?(x=w452) -> (x < 0?=w451:bool)
                  n221 = Format Into String(format string="%0.5e", w452) -> (resulting string=w453:string)  [unwired: 2 in, 1 out]
                  n222 = case shown="False" w451 {
                    tunnel: [w459 w463] -> w455
                    tunnel: w453 -> [w460 w462]
                    frame False {
                      n223 = Concatenate Strings(" " ("string"), w460, "\r\n") -> (w459:string)
                    }
                    frame True {
                      n224 = Concatenate Strings(w462, "\r\n") -> (w463:string)
                    }
                  }
                  n225 = Concatenate Strings(w456, w455) -> (w457:string)
                }
                n226 = Concatenate Strings(w423, w426, w427, w419) -> (w435:string)
                n227 = call "Write_File_Simple.vi"("append to file? (new file:F)"=FALSE, "character string"=w435, "file path"=w408) -> ()  [unwired: 2 out]
              }
              frame 2, Default {
                n228 = Subtract(x=w474, y=2) -> (x-y=w472:i32)
                n229 = Index Array(array=w465, index=w472) -> (element=w467:dbl)
                n230 = Format Into String(format string="%0.5e", w467) -> (resulting string=w469:string)  [unwired: 2 in, 1 out]
                n231 = Less Than 0?(x=w467) -> (x < 0?=w466:bool)
                n232 = case shown="False" w466 {
                  tunnel: [w477 w481] -> w468
                  tunnel: w469 -> [w478 w480]
                  frame False {
                    n233 = Concatenate Strings(" " ("string"), w478, "\r\n") -> (w477:string)
                  }
                  frame True {
                    n234 = Concatenate Strings(w480, "\r\n") -> (w481:string)
                  }
                }
                n235 = call "Write_File_Simple.vi"("append to file? (new file:F)"=TRUE, "character string"=w468, "file path"=w475) -> ()  [unwired: 2 out]
              }
            }
          }
        }
      }
    }
  }
